vi "PSU ON.vi"(8 "Error In":errorcluster, 11 "PSU Setting":T1={"Channel Name"="1", "Source Delay (Sec)"=0.5, "Measurement:Sense"=1008, "voltage level"=0.0, "voltage level range"=20.0, "current limit"=0.02, "current limit range"=0.02, "resource name"="PSU"} {"current limit range" format="%_6p"; "current limit" format="%_6p"; "voltage level range" format="%_6p"; "voltage level" format="%_6p"; "Measurement:Sense" items=["Local"=1008, "Remote"=1009]; "Source Delay (Sec)" format="%_6p"}) -> (0 "Error Out":errorcluster, 1 "Current Result (mA)":dbl, 2 "Volt Result":dbl, 3 "Result":dbl[](array[numeric]))   [LabVIEW 2018]
uses:
  PowerSupply4110/Type/SupplyConfig.ctl
panel:
  # "Einstellungen"
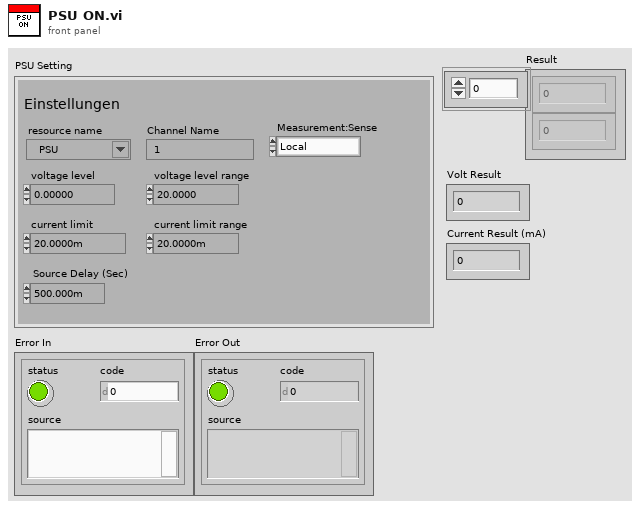
[diagram p1: front panel]
types:
  T1 = typedef "SupplyConfig.ctl" = cluster{"Channel Name":string, "Source Delay (Sec)":dbl, "Measurement:Sense":i32, "voltage level":dbl, "voltage level range":dbl, "current limit":dbl, "current limit range":dbl, "resource name":refnum<k15>}
  T2 = typedef "SupplyOutput.ctl" = cluster{"Current max":dbl, "Current min":dbl, "Voltage max":dbl, "Voltage min":dbl, "Voltage mean":dbl, "Current mean":dbl}
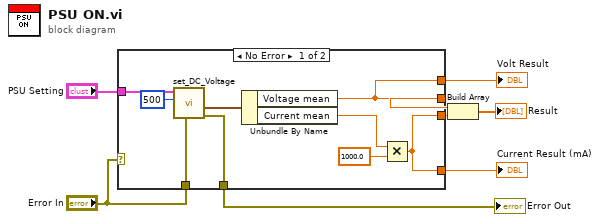
[diagram p0: block diagram]
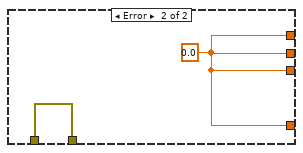
[diagram p2: hidden frame]
diagram:
  n1 = case shown="No Error" "Error In" {
    tunnel: "PSU Setting" -> [w17 _]
    tunnel: "Error In" -> [w16 w19]
    tunnel: [w15 w19] -> w7
    tunnel: [w13 w18] -> w4
    tunnel: [w10 w18] -> w5
    tunnel: [w13 w18] -> w2
    tunnel: [w10 w18] -> w1
    frame No Error {
      n2 = call "set_DC_Voltage.vi"("error in (no error)"=w16, "Messdauer/ms"=500, "Einstellungen"=w17) -> ("error out"=w15:errorcluster, "Supply Output"=w14:T2)  [unwired: 5 in, 2 out]
      n3 = Unbundle By Name(w14) -> ("Voltage mean"=w13:dbl, "Current mean"=w12:dbl)
      n4 = Multiply(x=w12, y=1000.0) -> (x*y=w10:dbl)
    }
    frame Error {
      w18 = 0.0 ("Voltage mean")
    }
  }
  "Error Out" <- w7
  "Current Result (mA)" <- w1
  "Volt Result" <- w2
  n5 = Build Array(w4, w5) -> (→"Result":dbl[])
